vi "Move Asset by ID.vi"(8 "error in (no error)":errorcluster, 10 "Physical Location":string, 11 "Asset ID":string) -> (0 "error out":errorcluster)   [LabVIEW 2024]
uses:
  Header--Combo Box.ctl
  POST (Buffer).vi
  Session.lvclass
  NI Skyline Configuration Library.lvlib
  NI Skyline Utilities.lvlib
panel:
  out "url":string
  out "body":string
  out "buffer":string
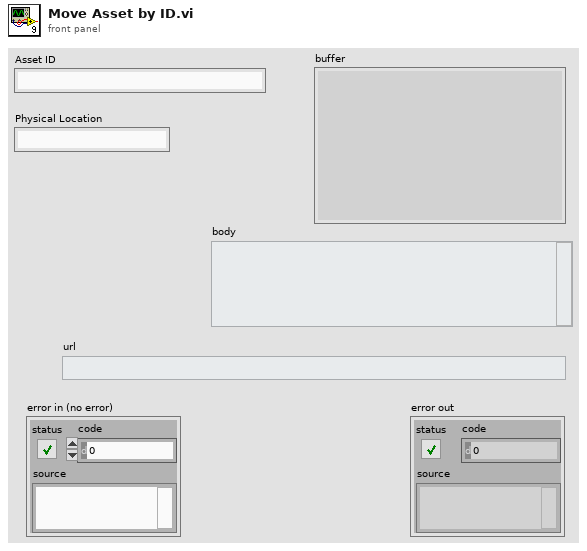
[diagram p1: front panel]
types:
  T1 = typedef "lib_NI_Advanced HTTP Client.lvlib/Session.lvclass/Header--Combo Box.ctl" = string
  T2 = typedef "NI Skyline Configuration Library.lvlib/Auto Configuration.ctl" = cluster{"id":string, "uri":string, "api key":string, "cert path":path, "owning file":path}
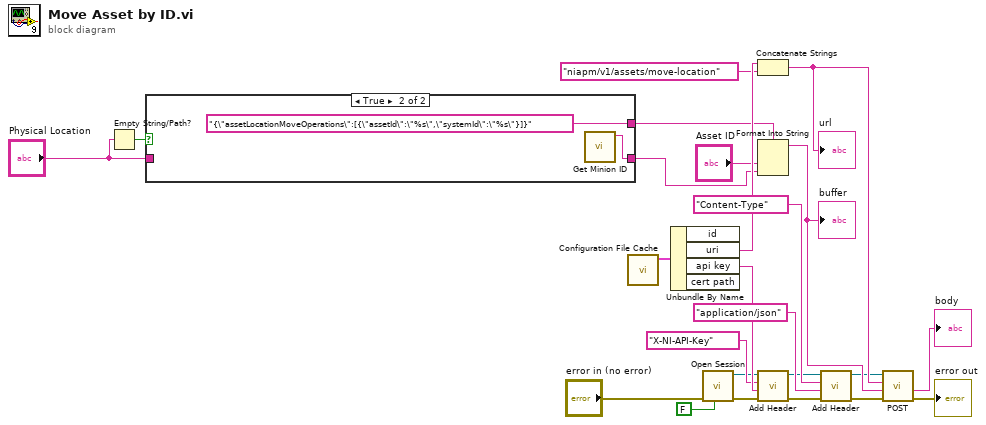
[diagram p0: block diagram]
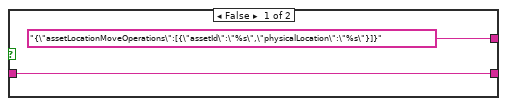
[diagram p2: hidden frame]
diagram:
  n1 = Empty String/Path?(string/path="Physical Location") -> (empty?=w4:bool)
  n2 = case shown="True" w4 {
    tunnel: ["{\"assetLocationMoveOperations\":[{\"assetId\":\"%s\",\"physicalLocation\":\"%s\"}]}" ("JSON") "{\"assetLocationMoveOperations\":[{\"assetId\":\"%s\",\"systemId\":\"%s\"}]}" ("JSON")] -> w3
    tunnel: [w26 w27] -> w2
    tunnel: "Physical Location" -> [w26 _]
    frame False {
    }
    frame True {
      n3 = call "Get Minion ID.vi"() -> ("minion id"=w27:string)  [unwired: 11 in]
    }
  }
  n4 = call "Configuration File Cache.vi"() -> ("HTTP configuration"=w17:T2)  [unwired: 10 in, 1 out]
  n5 = Unbundle By Name(w17) -> ("uri"=w22:string, "api key"=w21:string)  [unwired: 2 out]
  n6 = call "Open Session.vi"("verify server (T)"=FALSE, "error in"="error in (no error)") -> ("error out"=w19:errorcluster, "session"=w18:refnum<class "Session.lvclass">)  [unwired: 8 in]
  n7 = Concatenate Strings(w22, "niapm/v1/assets/move-location" ("url")) -> (w11:string)
  "url" <- w11
  n8 = Format Into String(format string=w3, "Asset ID", w2) -> (resulting string=w24:string)  [unwired: 2 in, 1 out]
  "buffer" <- w24
  n9 = call "Add Header.vi"("error in"=w19, "value"=w21, "header"=T1 "X-NI-API-Key", "session in"=w18) -> ("error out"=w7:errorcluster, "session out"=w8:refnum<class "Session.lvclass">)  [unwired: 6 in]
  n10 = call "Add Header.vi"("error in"=w7, "value"="application/json", "header"=T1 "Content-Type", "session in"=w8) -> ("error out"=w5:errorcluster, "session out"=w6:refnum<class "Session.lvclass">)  [unwired: 6 in]
  n11 = call-poly "POST.vi"("error in"=w5, "buffer"=w24, "url"=w11, "session in"=w6) -> ("error out"=→"error out":errorcluster, "body"=→"body":string)  [unwired: 3 in, 3 out]
